vi "v1h_get_NC_attrarray.vi"(3 "error in (no error)":errorcluster caption="错误输入（无错误）", 5 "refnum in":refnum<file>) -> (0 "error out":errorcluster, 1 "NC_attrarray":T1(array[cluster]) {"nc_type" items=["NC_NAT", "NC_BYTE", "NC_CHAR", "NC_SHORT", "NC_INT", "NC_FLOAT", "NC_DOUBLE"]}, 2 "refnum out":refnum<file>)   [LabVIEW 2016]
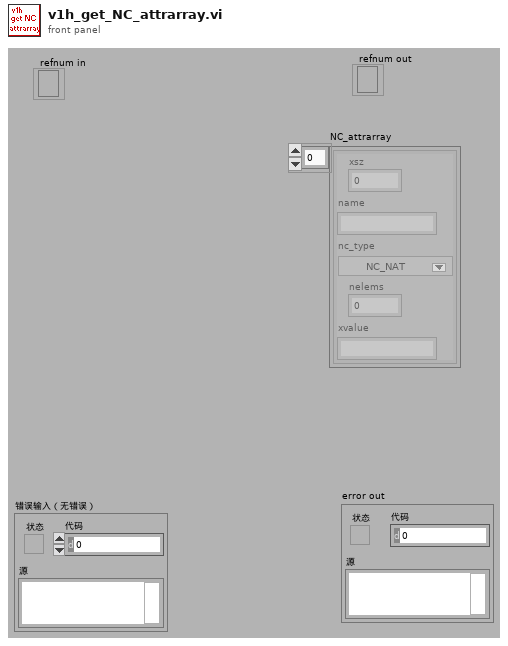
[diagram p1: front panel]
types:
  T1 = cluster{"xsz":u64, "name":string, "nc_type":u16, "nelems":u64, "xvalue":string}[]
  T2 = cluster{"xsz":u64, "name":string, "nc_type":u16, "nelems":u64, "xvalue":string}
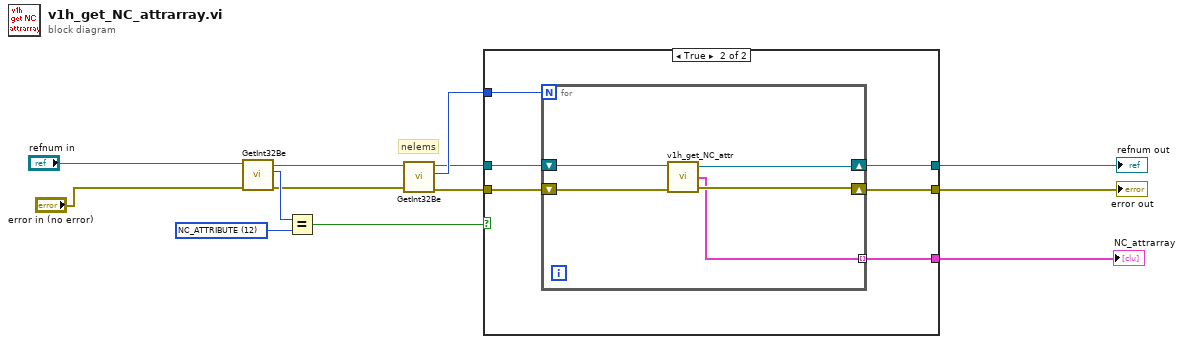
[diagram p0: block diagram]
diagram:
  w9 = u16 12 items=["NC_UNSPECIFIED"=0, "NC_BITFIELD"=7, "NC_STRING"=8, "NC_DIMENSION"=10, "NC_VARIABLE"=11, "NC_ATTRIBUTE"=12] ("NCtype")
  # "nelems"
  n1 = call "GetInt32Be.vi"("error in (no error)"="error in (no error)", "refnum in"="refnum in") -> ("error out"=w4:errorcluster, "int32"=w13:i32, "refnum out"=w8:refnum<file>)  [unwired: 3 out]
  n2 = Equal?(x=w13, y=w9) -> (x = y?=w5:bool)
  n3 = call "GetInt32Be.vi"("error in (no error)"=w4, "refnum in"=w8) -> ("error out"=w3:errorcluster, "int32"=w11:i32, "refnum out"=w10:refnum<file>)  [unwired: 3 out]
  n4 = case shown="True" w5 {
    tunnel: [_ w21] -> w1
    tunnel: [w15 w20] -> w12
    tunnel: w11 -> [_ w19]
    tunnel: w10 -> [w15 w18]
    tunnel: w3 -> [w14 w17]
    tunnel: [w14 w16] -> w6
    frame False {
    }
    frame True {
      n5 = for {
        N: w19 -> [_]
        shift-right: [w26] -> w20
        shift-left: w18 -> [w23]
        shift-right: [w24] -> w16
        shift-left: w17 -> [w25]
        tunnel: [w22] -> w21 mode=indexing
        n6 = call "v1h_get_NC_attr.vi"("errorin"=w25, "refnum in"=w23) -> ("error out"=w24:errorcluster, "NC_attr"=w22:T2, "refnum out"=w26:refnum<file>)  [unwired: 1 out]
      }
    }
  }
  "NC_attrarray" <- w1
  "refnum out" <- w12
  "error out" <- w6
